vi "PH_Calorimeter_USB.Subtract Offset.vi"(3 "Rate [Hz]":i32, 4 "Offset time [s]":dbl format="%.2f", 5 "DAQ Data [V]":dbl[](array[numeric]) format="%.2f") -> (1 "Offset [V]":dbl format="%0.2f", 2 "DAQ Data without Offset [V]":dbl[](array[numeric]) format="%.2f")   [LabVIEW 2014, in "PH_Calorimeter_USB.lvlib"]
doc: "This VI calculates the Offset from the data before the trigger went in and subtracts this value from all data. The result is given out at \"Data without offset\"."
uses:
  PH_Calorimeter_USB.lvlib
  <vilib>/Analysis/baseanly.llb/Mean (DBL).vi
  <vilib>/Analysis/NI_AALBase.lvlib
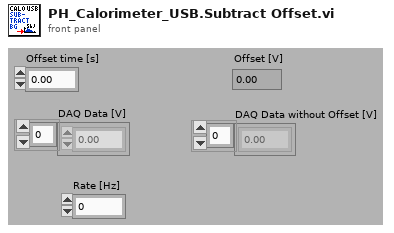
[diagram p1: front panel]
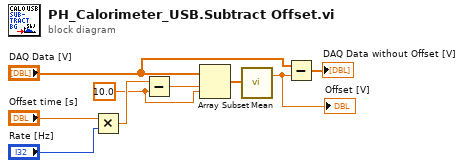
[diagram p0: block diagram]
diagram:
  w1 = 10.0 ("y")
  n1 = Multiply(x="Offset time [s]", y="Rate [Hz]") -> (x*y=w3:dbl)
  n2 = Subtract(x=w3, y=w1) -> (x-y=w2:dbl)
  n3 = Array Subset(array="DAQ Data [V]", index=w2, length=w1) -> (w8:dbl[])
  n4 = call-poly <vilib>:"Mean.vi"("X"=w8) -> ("mean"=w7:dbl)  [unwired: 1 out]
  "Offset [V]" <- w7
  n5 = Subtract(x="DAQ Data [V]", y=w7) -> (x-y=→"DAQ Data without Offset [V]":dbl[])
